vi "Ark Dino Leveler.vi"(8 "error in (no error)":errorcluster) -> (0 "error out":errorcluster)   [LabVIEW 2023]
uses:
  CTLs/Dump Stat.ctl
  <vilib>/Utility/config.llb/Config Data RefNum.ctl
  eb7943ba-f707-43d5-9dff-d1005f5da418.vi
  <vilib>/Utility/config.llb/Write Key (I32).vi
  <vilib>/Utility/inputDevices.llb/closeKeyboard.vi
  <vilib>/Utility/inputDevices.llb/closeMouse.vi
  <userlib>/_MGI/Application Control/MGI Gray if/MGI Gray if False.vi
  <vilib>/Utility/inputDevices.llb/keyboardAcquire.vi
  FaKI State Machine/FaKI State Machine.lvlib
  <vilib>/Utility/config.llb/NI_LVConfig.lvlib
panel:
  out "Application Hotkey":string
  in  "Delete Preset":bool
  in  "Select Monitor":i32=1 min=1 max=6
  in  "Start/Stop":bool
  in  "Dump Stat":T1
  out "Levels Remaining":i32
  in  "Levels Available":i32=85 min=0 max=1000
  in  "Save Preset":bool
  in  "Preset Name":string(combo)
  in  "No Oxy Stat?":bool
  in  "Levels":T2 {"HP" min=0 max=200; "Stamina" min=0 max=200; "Oxygen" min=0 max=200; "Food" min=0 max=200; "Weight" min=0 max=200; "Melee" min=0 max=200; "Speed" min=0 max=200}
  in  "Exit":bool
  # "(all remaining points go here)"
  # "(Golems, water tames, etc)"
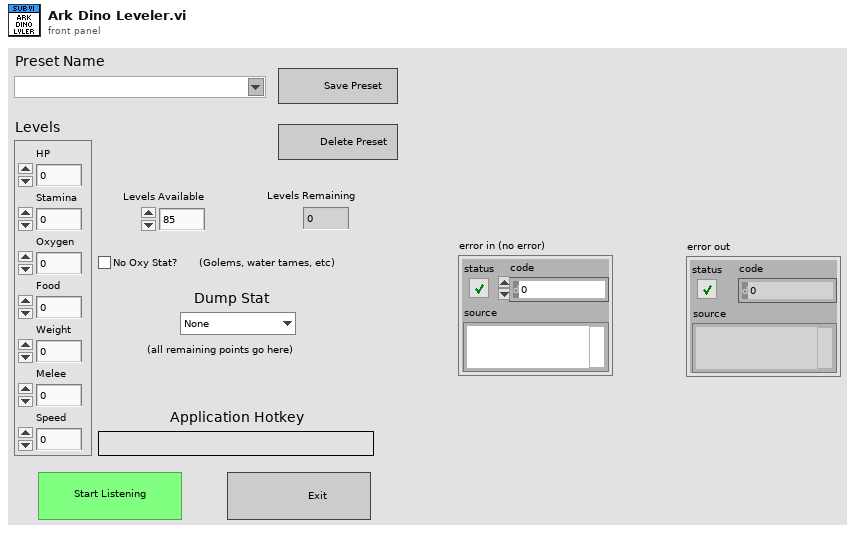
[diagram p1: front panel]
types:
  T1 = typedef "Dump Stat.ctl" = enum16{"None", "HP", "Stamina", "Oxygen", "Food", "Weight", "Melee", "Speed"}
  T2 = cluster{"HP":i32, "Stamina":i32, "Oxygen":i32, "Food":i32, "Weight":i32, "Melee":i32, "Speed":i32}
  T3 = enum8{"Enabled", "Disabled", "Disabled and Grayed Out"}
  T4 = enum32{"Invalid", "Standard", "Closed", "Hidden", "Minimized", "Maximized"}
  T5 = enum32{"invalid app kind", "Development System", "Run Time System", "Student Edition", "Embedded LabVIEW", "Evaluation", "Custom"}
  T6 = typedef "NI_LVConfig.lvlib/Config Data RefNum.ctl" = refnum<k1>
  T7 = cluster{"Core":cluster{"Current VI Reference":refnum<vi>, "Close Panel on Exit?":bool}, "Mouse":refnum<k1>, "Keyboard":refnum<k1>, "Config":T6, "Hotkey":enum16{"0", "1", "2", "3", "4", "5", "6", "7", "8", "9", "A", "B", "C", "D", "E", "F", "G", "H", "I", "J", "K", "L", "M", "N", "O", "P", "Q", "R", "S", "T", "U", "V", "W", "X", "Y", "Z", "F1", "F2", "F3", "F4", "F5", "F6", "F7", "F8", "F9", "F10", "F11", "F12", "F13", "F14", "F15", "ADD", "BACK", "BACKSLASH", "CAPITAL", "COMMA", "DECIMAL", "DELETE", "DIVIDE", "DOWN", "END", "EQUALS", "ESCAPE", "GRAVE (`)", "HOME", "INSERT", "LBRACKET", "LCONTROL", "LEFT", "L ALT", "LSHIFT", "LWIN", "MINUS", "MULTIPLY", "NEXT", "NUMLOCK", "NUMPAD_0", "NUMPAD_1", "NUMPAD_2", "NUMPAD_3", "NUMPAD_4", "NUMPAD_5", "NUMPAD_6", "NUMPAD_7", "NUMPAD_8", "NUMPAD_9", "PAUSE", "PERIOD", "PRIOR (PG UP)", "RBRACKET", "RCONTROL", "RETURN", "RIGHT", "R ALT", "RSHIFT", "RWIN", "SCROLL", "SEMICOLON", "SLASH", "SPACE", "SUBTRACT", "TAB", "UP", "ENTER (num pad)", "' (quote)"}[], "Res":cluster{"V":i16, "H":i16}[]}
  T8 = enum16{"0", "1", "2", "3", "4", "5", "6", "7", "8", "9", "A", "B", "C", "D", "E", "F", "G", "H", "I", "J", "K", "L", "M", "N", "O", "P", "Q", "R", "S", "T", "U", "V", "W", "X", "Y", "Z", "F1", "F2", "F3", "F4", "F5", "F6", "F7", "F8", "F9", "F10", "F11", "F12", "F13", "F14", "F15", "ADD", "BACK", "BACKSLASH", "CAPITAL", "COMMA", "DECIMAL", "DELETE", "DIVIDE", "DOWN", "END", "EQUALS", "ESCAPE", "GRAVE (`)", "HOME", "INSERT", "LBRACKET", "LCONTROL", "LEFT", "L ALT", "LSHIFT", "LWIN", "MINUS", "MULTIPLY", "NEXT", "NUMLOCK", "NUMPAD_0", "NUMPAD_1", "NUMPAD_2", "NUMPAD_3", "NUMPAD_4", "NUMPAD_5", "NUMPAD_6", "NUMPAD_7", "NUMPAD_8", "NUMPAD_9", "PAUSE", "PERIOD", "PRIOR (PG UP)", "RBRACKET", "RCONTROL", "RETURN", "RIGHT", "R ALT", "RSHIFT", "RWIN", "SCROLL", "SEMICOLON", "SLASH", "SPACE", "SUBTRACT", "TAB", "UP", "ENTER (num pad)", "' (quote)"}[]
  T9 = cluster{"Current VI Reference":refnum<vi>, "Close Panel on Exit?":bool}
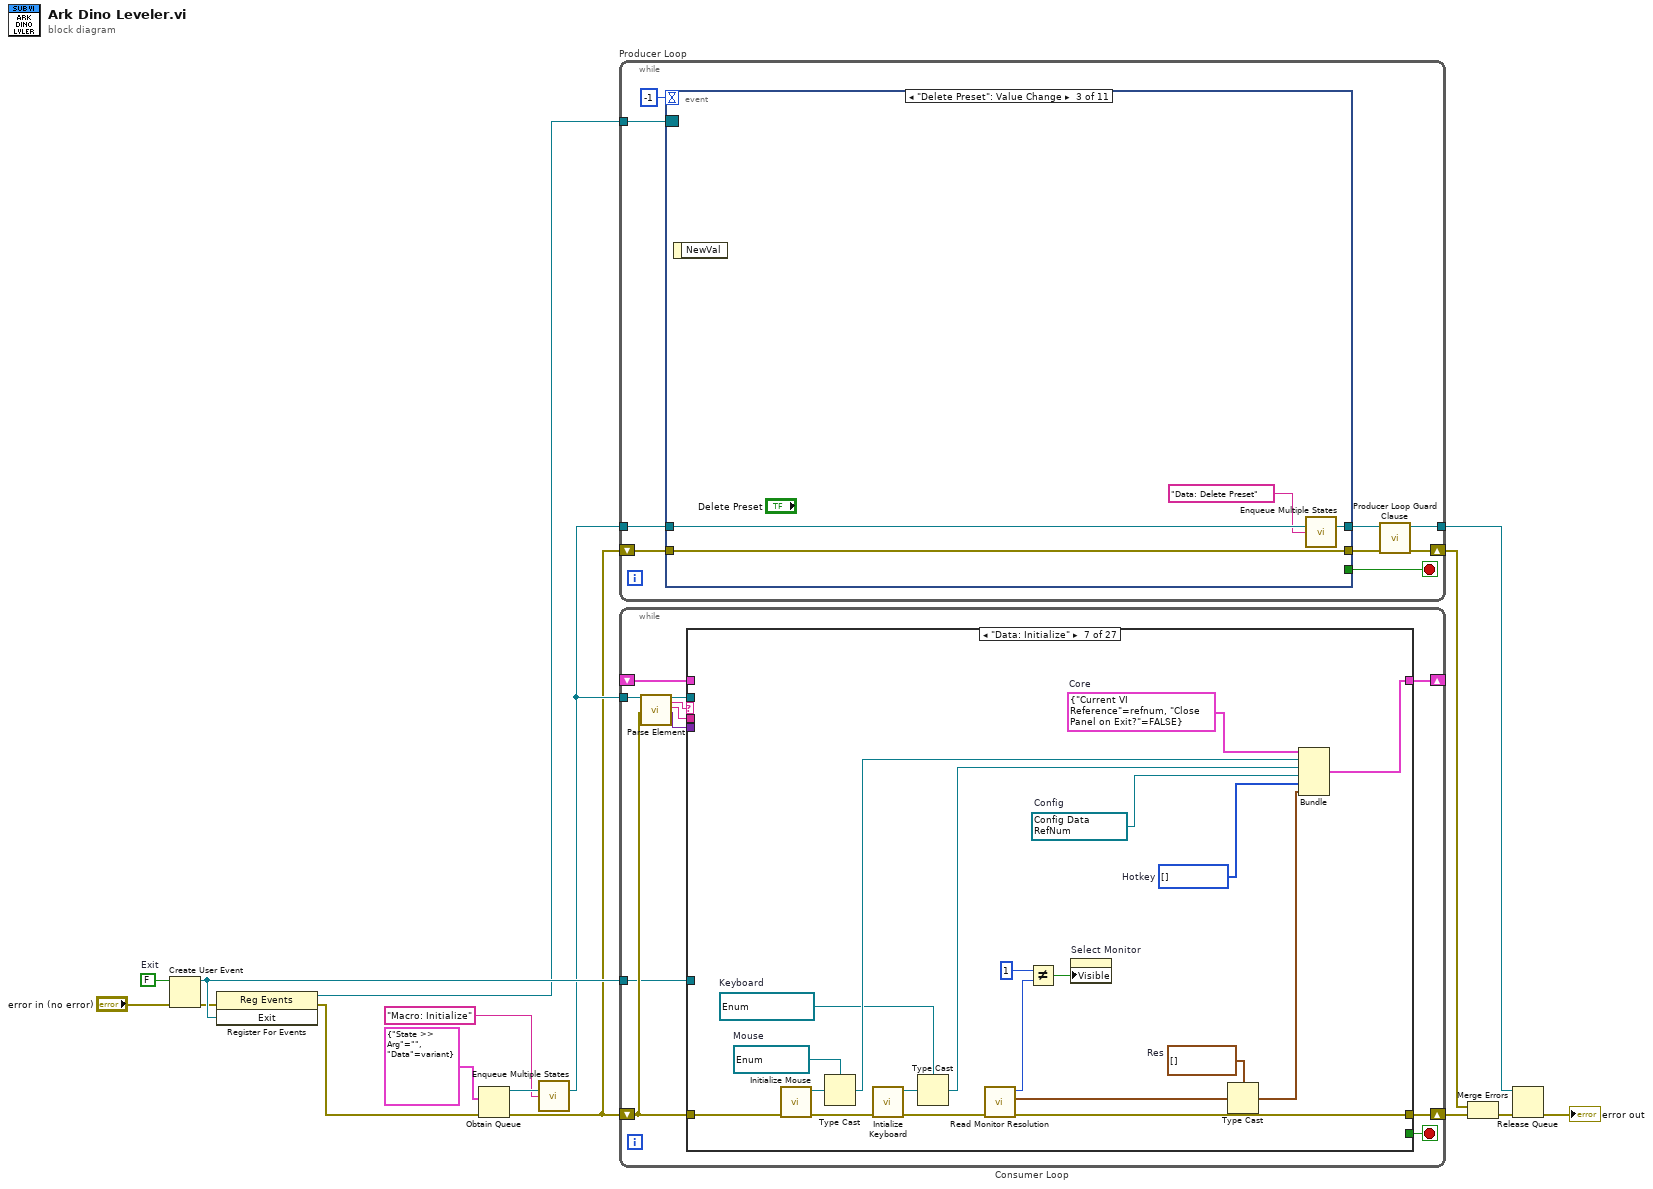
[diagram p0: block diagram]
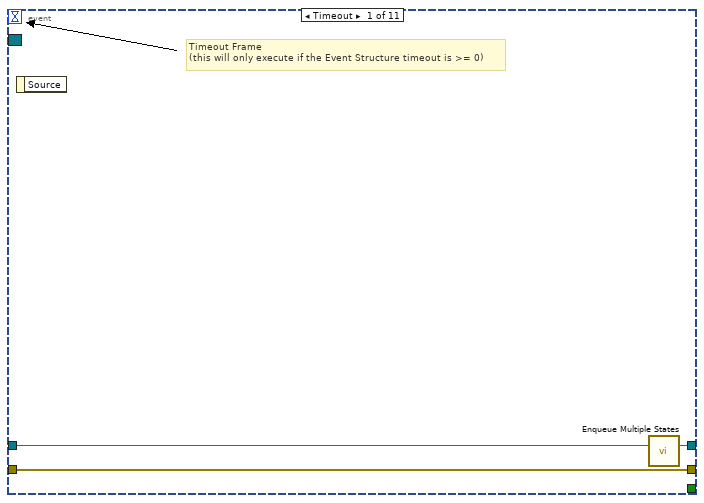
[diagram p2: hidden frame]
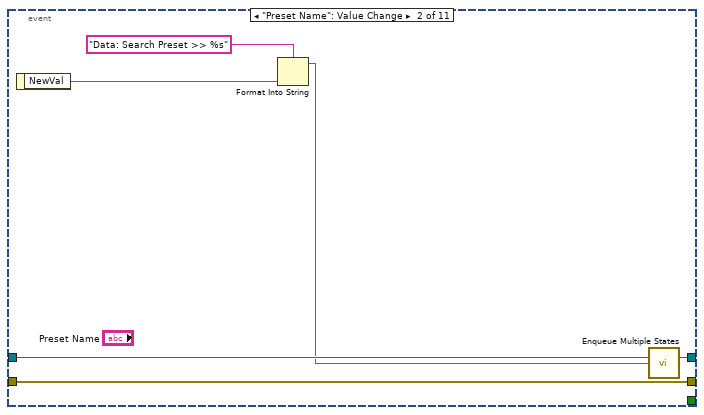
[diagram p3: hidden frame]
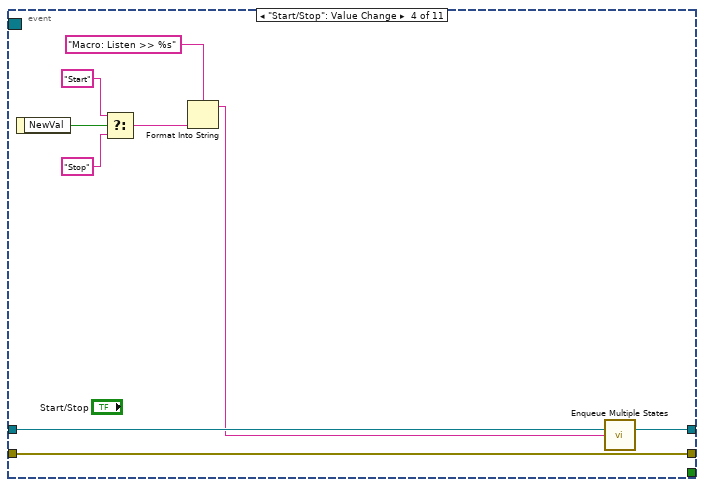
[diagram p4: hidden frame]
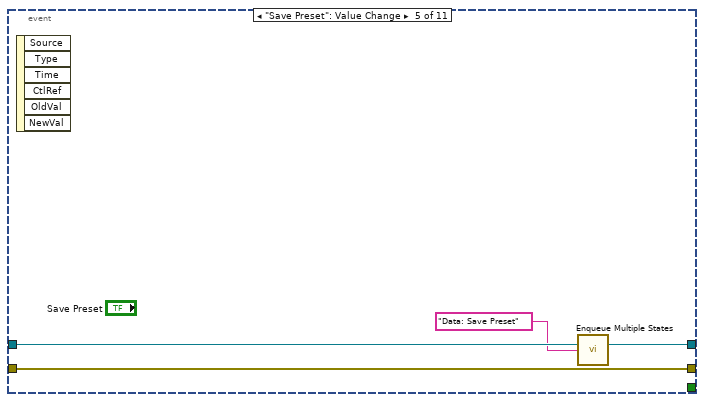
[diagram p5: hidden frame]
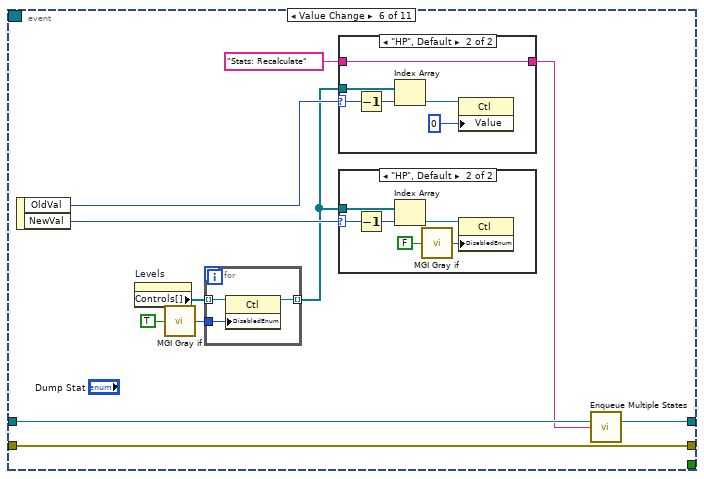
[diagram p6: hidden frame]
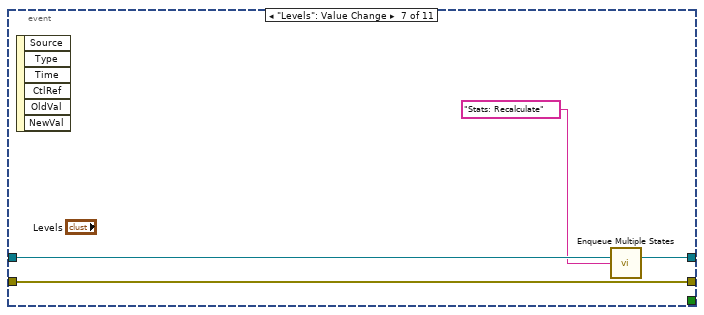
[diagram p9: hidden frame]
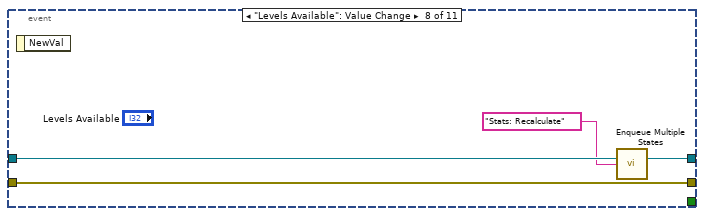
[diagram p10: hidden frame]
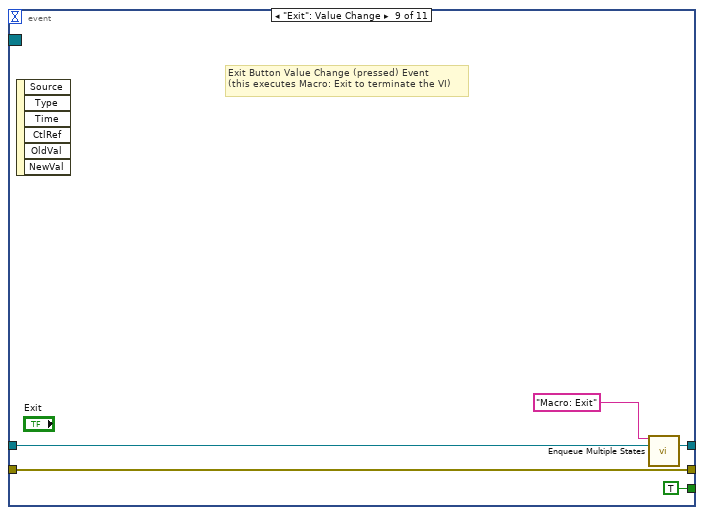
[diagram p11: hidden frame]
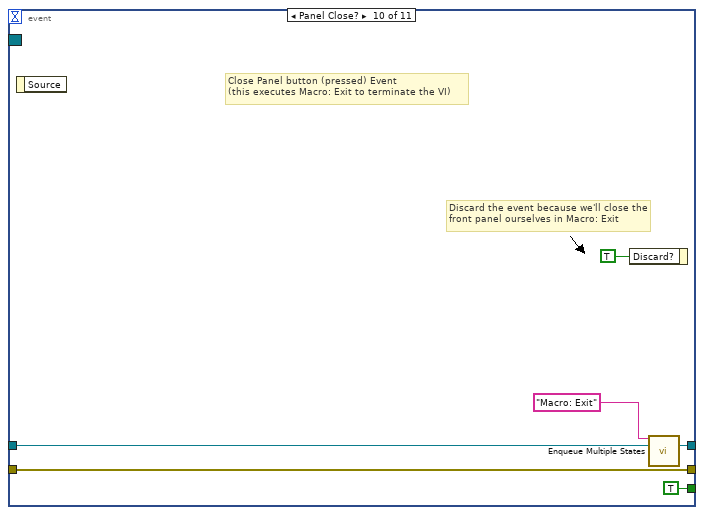
[diagram p12: hidden frame]
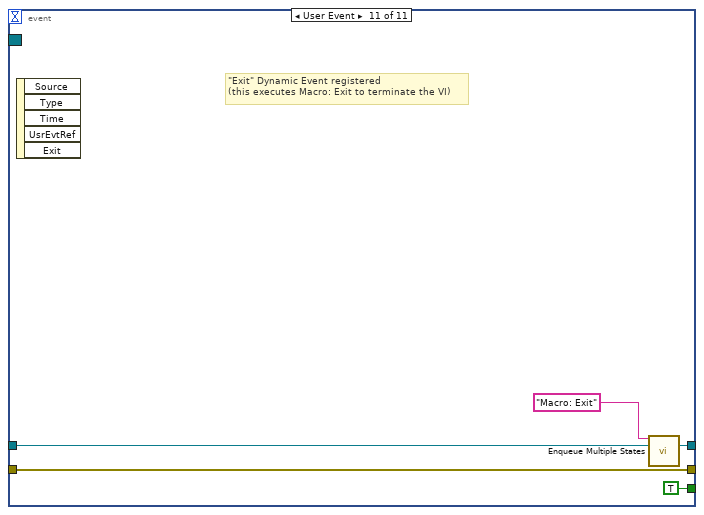
[diagram p13: hidden frame]
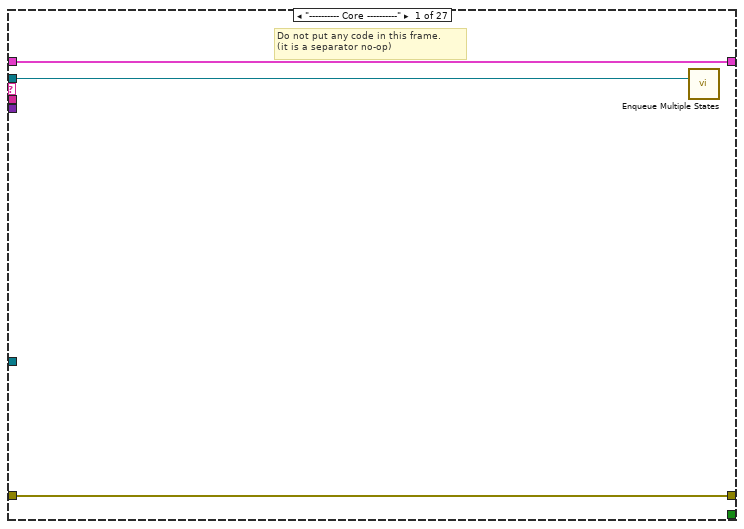
[diagram p14: hidden frame]
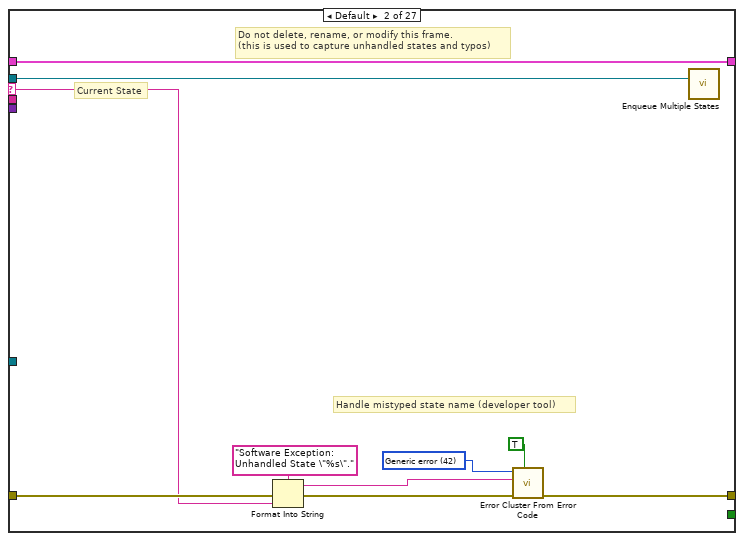
[diagram p15: hidden frame]
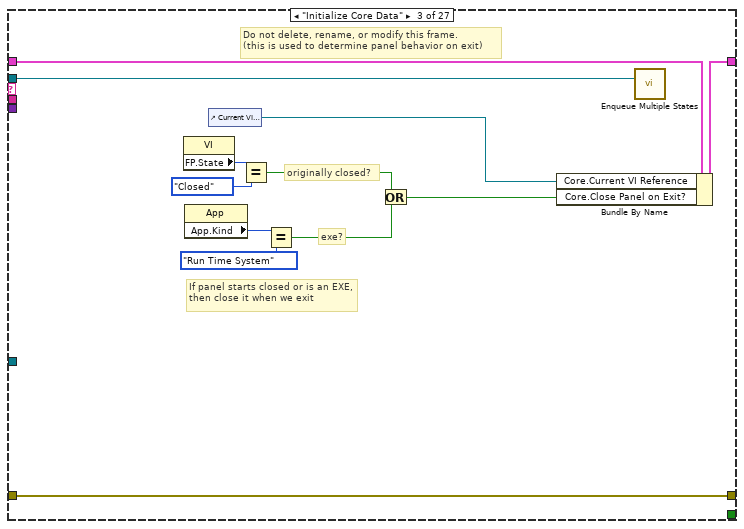
[diagram p16: hidden frame]
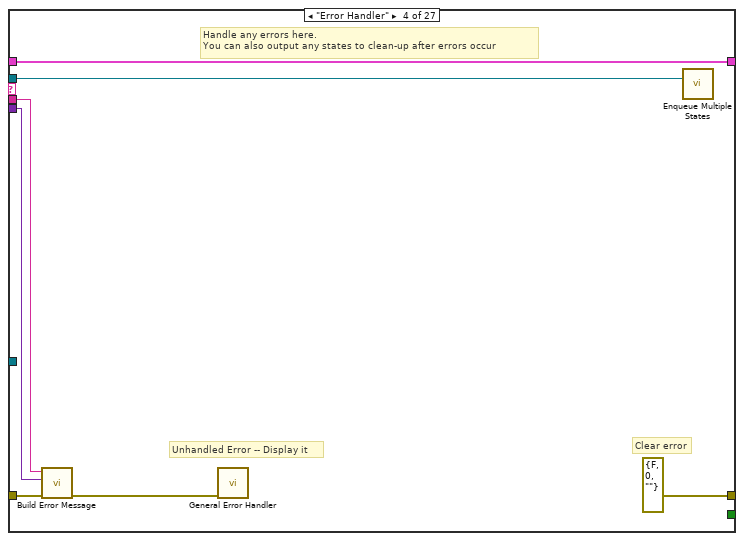
[diagram p17: hidden frame]
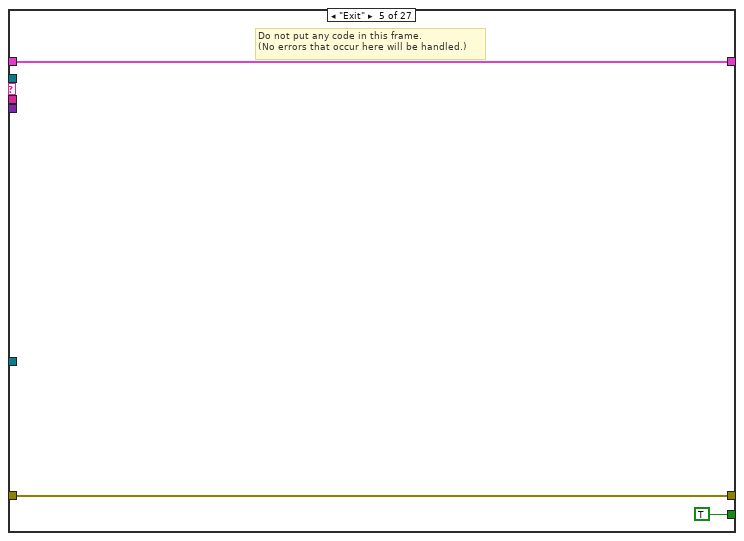
[diagram p18: hidden frame]
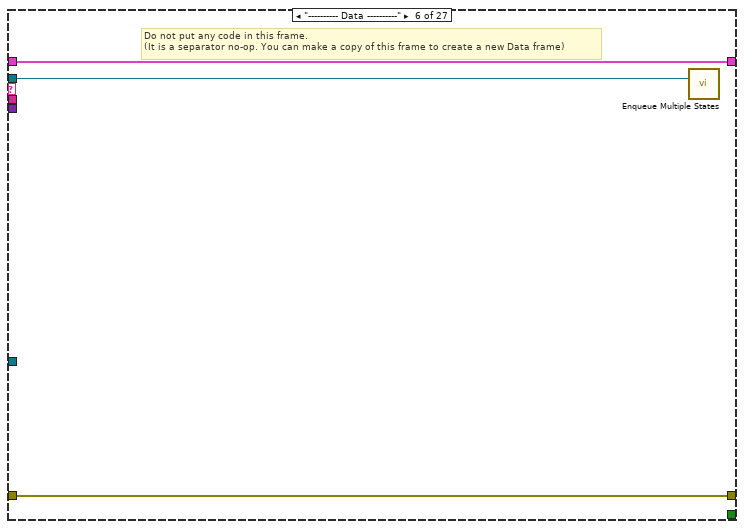
[diagram p19: hidden frame]
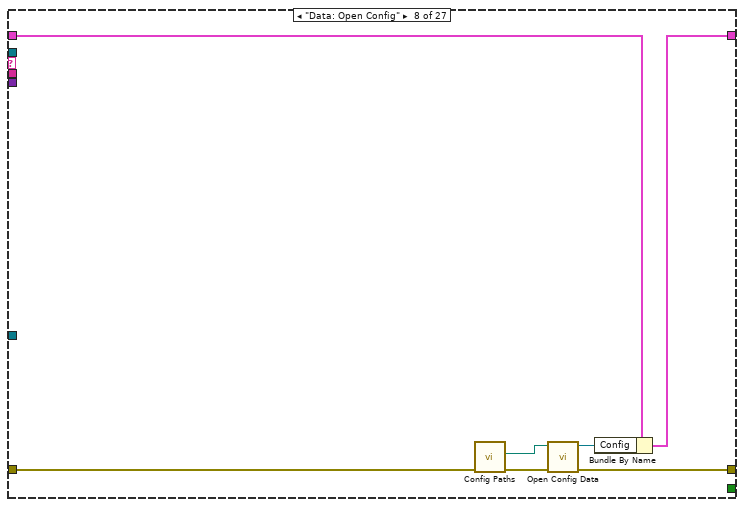
[diagram p20: hidden frame]
diagram:
  w13 = FALSE  # Exit
  n1 = Create User Event(user event datatype=w13, error in="error in (no error)") -> (user event=w16:refnum<user-event>, error out=w12:errorcluster)
  n2 = register-events(error in=w12, w16) -> (reference out=w15:refnum<event-registration>, error out=w14:errorcluster)  [unwired: 1 in]
  n3 = Obtain Queue(element data type=cluster{"State >> Arg":string, "Data":variant} {"State >> Arg"="", "Data"=variant}, error in (no error)=w14) -> (queue out=w6:refnum<queue>, error out=w3:errorcluster)  [unwired: 3 in, 1 out]
  n4 = call "Enqueue Multiple States.vi"("queue in"=w6, "State(s) at Back"="Macro: Initialize") -> ("queue out"=w7:refnum<queue>)  [unwired: 13 in]
  n5 = while "Producer Loop" {
    shift-right: [w20] -> w9
    shift-left: w3 -> [w25]
    tunnel: w15 -> [w17]
    tunnel: w7 -> [w23]
    tunnel: [w18] -> w11
    stop <- w22 stop-if-true
    n6 = event shown="[2] \"Delete Preset\": Value Change" {
      selector: w17 -> [_ _ _ _ _ _ _ _ _ _ _]
      dyn-events: _ -> [_ _ _ _ _ _ _ _ _ _ _]
      timeout: -1 ("Timeout") -> [_ _ _ _ _ _ _ _ _ _ _]
      tunnel: [w26 w32 w36 w47 w51 w62 w82 w86 w91 w97 w102] -> w21
      tunnel: w25 -> [w26 w32 w36 w47 w51 w62 w82 w86 w91 w97 w102]
      tunnel: w23 -> [w27 w33 w37 w43 w50 w53 w81 w85 w90 w94 w100]
      tunnel: [w28 w34 w38 w39 w49 w54 w80 w84 w88 w93 w99] -> w19
      tunnel: [_ _ _ _ _ _ _ _ TRUE TRUE TRUE] -> w22
      event Timeout {
        # "Timeout Frame\n(this will only execute if the Event Structure timeout is >= 0)"
        n7 = event-data() -> ()  [unwired: 1 in, 1 out]
        n8 = call "Enqueue Multiple States.vi"("queue in"=w27) -> ("queue out"=w28:refnum<queue>)  [unwired: 14 in]
      }
      event "Preset Name": Value Change {
        n9 = event-data() -> ("NewVal"=w30:string)  [unwired: 1 in]
        n10 = Format Into String(format string="Data: Search Preset >> %s" ("State(s) at Back"), w30) -> (resulting string=w29:string)  [unwired: 2 in, 1 out]
        n11 = call "Enqueue Multiple States.vi"("queue in"=w33, "State(s) at Back"=w29) -> ("queue out"=w34:refnum<queue>)  [unwired: 13 in]
      }
      event "Delete Preset": Value Change {
        n12 = event-data() -> ()  [unwired: 1 in, 1 out]
        n13 = call "Enqueue Multiple States.vi"("queue in"=w37, "State(s) at Back"="Data: Delete Preset") -> ("queue out"=w38:refnum<queue>)  [unwired: 13 in]
      }
      event "Start/Stop": Value Change {
        n14 = event-data() -> ("NewVal"=w44:bool)  [unwired: 1 in]
        n15 = Select(t="Start", s=w44, f="Stop") -> (s? t:f=w41:string)
        n16 = Format Into String(format string="Macro: Listen >> %s", w41) -> (resulting string=w40:string)  [unwired: 2 in, 1 out]
        n17 = call "Enqueue Multiple States.vi"("queue in"=w43, "State(s) at Back"=w40) -> ("queue out"=w39:refnum<queue>)  [unwired: 13 in]
      }
      event "Save Preset": Value Change {
        n18 = event-data() -> ()  [unwired: 1 in, 6 out]
        n19 = call "Enqueue Multiple States.vi"("queue in"=w50, "State(s) at Back"="Data: Save Preset") -> ("queue out"=w49:refnum<queue>)  [unwired: 13 in]
      }
      event Value Change {
        n20 = event-data() -> ("OldVal"=w57:T1, "NewVal"=w61:T1)  [unwired: 1 in]
        n21 = property on="Levels" class="Clust (strict)"() -> ("Controls[]"=w58:refnum<vi>[])  [unwired: 2 in, 2 out]
        n22 = call-poly <userlib>:"MGI Gray if.vi"("Boolean"=TRUE) -> ("Disabled"=w60:T3)
        n23 = for {
          tunnel: w58 -> [w72] mode=indexing
          tunnel: w60 -> [w71]
          tunnel: [w70] -> w56 mode=indexing
          n24 = property class="Ctl"(reference=w72, "DisabledEnum"=w71) -> (reference out=w70:refnum<vi>)  [unwired: 1 in, 1 out]
        }
        n25 = case shown="\"HP\", Default" w57 {
          selector: w57 -> [_ w69]
          tunnel: w56 -> [_ w68]
          tunnel: "Stats: Recalculate" -> [w63 w64]
          tunnel: [w63 w64] -> w52
          frame "None" {
          }
          frame "HP", Default {
            n26 = Decrement(x=w69) -> (x-1=w67:T1)
            n27 = Index Array(array=w68, index=w67) -> (element=w66:refnum<vi>)
            n28 = property class="Ctl"(reference=w66, "Value"=0 ("Select Monitor")) -> ()  [unwired: 1 in, 2 out]
          }
        }
        n29 = case shown="\"HP\", Default" w61 {
          selector: w61 -> [_ w78]
          tunnel: w56 -> [_ w75]
          frame "None" {
          }
          frame "HP", Default {
            n30 = Decrement(x=w78) -> (x-1=w74:T1)
            n31 = Index Array(array=w75, index=w74) -> (element=w73:refnum<vi>)
            n32 = call-poly <userlib>:"MGI Gray if.vi"("Boolean"=FALSE) -> ("Disabled"=w76:T3)
            n33 = property class="Ctl"(reference=w73, "DisabledEnum"=w76) -> ()  [unwired: 1 in, 2 out]
          }
        }
        n34 = call "Enqueue Multiple States.vi"("queue in"=w53, "State(s) at Back"=w52) -> ("queue out"=w54:refnum<queue>)  [unwired: 13 in]
      }
      event "Levels": Value Change {
        n35 = event-data() -> ()  [unwired: 1 in, 6 out]
        n36 = call "Enqueue Multiple States.vi"("queue in"=w81, "State(s) at Back"="Stats: Recalculate") -> ("queue out"=w80:refnum<queue>)  [unwired: 13 in]
      }
      event "Levels Available": Value Change {
        n37 = event-data() -> ()  [unwired: 1 in, 1 out]
        n38 = call "Enqueue Multiple States.vi"("queue in"=w85, "State(s) at Back"="Stats: Recalculate") -> ("queue out"=w84:refnum<queue>)  [unwired: 13 in]
      }
      event "Exit": Value Change {
        # "Exit Button Value Change (pressed) Event\n(this executes Macro: Exit to terminate the VI)"
        n39 = event-data() -> ()  [unwired: 1 in, 6 out]
        n40 = call "Enqueue Multiple States.vi"("State(s) at Front"="Macro: Exit", "queue in"=w90) -> ("queue out"=w88:refnum<queue>)  [unwired: 13 in]
      }
      event Panel Close? {
        # "Discard the event because we'll close the front panel ourselves in Macro: Exit"
        # "Close Panel button (pressed) Event\n(this executes Macro: Exit to terminate the VI)"
        n41 = event-data() -> ()  [unwired: 1 in, 1 out]
        n42 = event-data("Discard?"=TRUE) -> ()  [unwired: 1 in, 1 out]
        n43 = call "Enqueue Multiple States.vi"("State(s) at Front"="Macro: Exit", "queue in"=w94) -> ("queue out"=w93:refnum<queue>)  [unwired: 13 in]
      }
      event User Event {
        # "\"Exit\" Dynamic Event registered\n(this executes Macro: Exit to terminate the VI)"
        n44 = event-data() -> ()  [unwired: 1 in, 5 out]
        n45 = call "Enqueue Multiple States.vi"("State(s) at Front"="Macro: Exit", "queue in"=w100) -> ("queue out"=w99:refnum<queue>)  [unwired: 13 in]
      }
    }
    n46 = call "Producer Loop Guard Clause.vi"("error in (no error)"=w21, "queue in"=w19) -> ("error out"=w20:errorcluster, "queue out"=w18:refnum<queue>)  [unwired: 8 in]
  }
  n47 = while "Consumer Loop" {
    shift-right: [w110] -> _
    shift-left: _ -> [w109]
    shift-right: [w113] -> w8
    shift-left: w3 -> [w112]
    tunnel: w7 -> [w108]
    tunnel: w16 -> [w103]
    stop <- w111 stop-if-true
    n48 = call "Parse Element.vi"("queue in"=w108, "error in (no error)"=w112) -> ("queue out"=w107:refnum<queue>, "State"=w106:string, "Arg"=w105:string, "Data"=w104:variant)  [unwired: 14 in]
    n49 = case shown="\"Data: Initialize\"" w106 {
      selector: w106 -> [_ w118 _ _ _ _ _ _ _ _ _ _ _ _ _ _ _ _ _ _ _ _ _ _ _ _ _]
      tunnel: w107 -> [w114 w117 w127 w143 _ w149 _ _ w181 _ w202 _ _ w297 w300 w312 w316 w325 _ w407 w417 w420 w427 w434 w440 w450 _]
      tunnel: w105 -> [_ _ _ w139 _ _ _ _ _ w185 _ _ _ _ _ _ w317 w326 _ _ _ _ w426 _ _ _ _]
      tunnel: w109 -> [w115 w120 w133 w144 w147 w150 _ w178 w182 w190 w206 w256 w280 w294 w301 w304 w318 w328 w397 w416 w418 w422 w428 w438 w441 w451 w456]
      tunnel: [w116 w125 w138 errorcluster {"status"=FALSE, "code"=0, "source"=""} ("error out") w148 w151 w160 w175 w179 w183 w204 w253 w278 w295 w302 w310 w319 w329 w399 w413 w419 w423 w425 w439 w442 w452 w458] -> w113
      tunnel: w112 -> [w116 w124 w138 w142 w148 w151 w170 w174 w180 w191 w213 w263 w281 w299 w302 w311 w320 w330 w400 w414 w419 w423 w425 w439 w442 w452 w459]
      tunnel: [_ _ _ _ TRUE _ _ _ _ _ _ _ _ _ _ _ _ _ _ _ _ _ _ _ _ _ _] -> w111
      tunnel: [w115 w120 w137 w144 w147 w150 w166 w177 w182 w190 w203 w258 w280 w294 w301 w303 w318 w328 w397 w416 w418 w422 w428 w438 w441 w451 w456] -> w110
      tunnel: w104 -> [_ _ _ w140 _ _ _ _ _ _ _ _ _ _ _ _ _ _ _ _ _ _ _ _ _ _ _]
      tunnel: w103 -> [_ _ _ _ _ _ _ _ _ _ _ _ _ _ _ _ _ _ _ _ _ _ _ _ _ _ _]
      frame "---------- Core ----------" {
        # "Do not put any code in this frame.\n(it is a separator no-op)"
        n50 = call "Enqueue Multiple States.vi"("queue in"=w114) -> ()  [unwired: 14 in, 1 out]
      }
      frame Default {
        w122 = 42 items=["No error", "Argument error", "Memory is full", "Out of zone", "End of file", "File already open", "Generic file I/O error", "File not found", "File permission error", "Disk is full", "Duplicate path", "Too many files open", "System feature not enabled", "Resource file not found", "Cannot add resource", "Resource not found", "Image not found", "Image memory error", "Pen does not exist", "Config type invalid", "Config token not found", "Config parse error", "Config memory error", "Bad external code format", "Bad external code offset", "External code not present", "Null window", "Destroy window error", "Null menu", "Print aborted", "Bad print record", "Print driver error", "Windows error during printing", "Memory error during printing", "Print dialog error", "Generic print error", "Invalid device refnum", "Device not found", "Device parameter error", "Device unit error", "Cannot open device", "Device call aborted", "Generic error", "Cancelled by user", "Object ID too low", "Object ID too high", "Object not in heap", "Unknown heap", "Unknown object (invalid DefProc)", "Unknown object (DefProc not in table)", "Message out of range", "Invalid (null) method", "Unknown message", "Manager call not supported", "Bad address", "Network operation in progress", "Network operation timed out", "Connection is busy", "Network attribute not supported", "Network error", "Address in use", "System out of memory", "Connection aborted", "Connection refused", "Not connected", "Already connected", "Connection closed", "Initialization error (interapplication manager)", "Bad occurrence", "Wait on unbound occurrence handler", "Occurrence queue overflow", "Datalog type conflict", "Unused", "Unrecognized type (interapplication manager)", "Memory corrupt", "Failed to make temporary DLL", "Old CIN version", "Drag socket not found", "Failed to load drop-object", "Failed to register OLE object", "Failed to release OLE object", "Format specifier type mismatch", "Unknown format specifier", "Too few format specifiers", "Too many format specifiers", "Scan failed", "Newer CIN version", "Error converting to variant", "Runtime menu error", "Password tampered", "Variant attribute not found", "Incompatible variant data type", "Event data is not available", "Event Store is not present", "Occurrence is not found", "Event Queue is not created", "Event info is not available", "Refnum passed is NULL", "Error retrieving Class GUID", "Error retrieving CoClass GUID", "Error retrieving TypeLib GUID.", "Bad built application magic bytes.", "Specific driver is different from the specific driver associated with the Logical Name.", "There is no session opened to the class driver.", "Max Error", "MAX - Error with config objects", "MAX - Error loading configuration", "MAX - Group not supported"]
        # "Current State"
        # "Do not delete, rename, or modify this frame.\n(this is used to capture unhandled states and typos)"
        # "Handle mistyped state name (developer tool)"
        n51 = Format Into String(format string="Software Exception: Unhandled State \"%s\"." ("message"), error in=w124, w118) -> (resulting string=w121:string, error out=w126:errorcluster)  [unwired: 1 in]
        n52 = call <vilib>:"Error Cluster From Error Code.vi"("show call chain? (False)"=TRUE, "error in (no error)"=w126, "error message (\"\")"=w121, "error code (0)"=w122) -> ("error out"=w125:errorcluster)  [unwired: 5 in]
        n53 = call "Enqueue Multiple States.vi"("queue in"=w117) -> ()  [unwired: 14 in, 1 out]
      }
      frame "Initialize Core Data" {
        # "Do not delete, rename, or modify this frame.\n(this is used to determine panel behavior on exit)"
        # "originally closed?"
        # "exe?"
        # "If panel starts closed or is an EXE, then close it when we exit"
        n54 = property class="VI"() -> ("FP.State"=w130:T4)  [unwired: 2 in, 2 out]
        n55 = property class="App"() -> ("App.Kind"=w136:T5)  [unwired: 2 in, 2 out]
        n56 = control-ref of="Current VI Reference"() -> (w131:refnum<vi>)
        n57 = Equal?(x=w130, y=T4."Closed" ("Front Panel Window:State")) -> (x = y?=w128:bool)
        n58 = Equal?(x=w136, y=T5."Run Time System" ("Application:Kind")) -> (x = y?=w134:bool)
        n59 = Or(x=w128, y=w134) -> (x .or. y?=w132:bool)
        n60 = Bundle By Name(cluster=w133, "Core.Current VI Reference"=w131, "Core.Close Panel on Exit?"=w132) -> (w137:T7)
        n61 = call "Enqueue Multiple States.vi"("queue in"=w127) -> ()  [unwired: 14 in, 1 out]
      }
      frame "Error Handler" {
        # "Unhandled Error -- Display it"
        # "Handle any errors here.\nYou can also output any states to clean-up after errors occur"
        # "Clear error"
        n62 = call "Build Error Message.vi"("error in (no error)"=w142, "Data"=w140, "Arg"=w139) -> ("error out"=w141:errorcluster)  [unwired: 8 in]
        n63 = call <vilib>:"General Error Handler.vi"("error in (no error)"=w141) -> ()  [unwired: 10 in, 5 out]
        n64 = call "Enqueue Multiple States.vi"("queue in"=w143) -> ()  [unwired: 14 in, 1 out]
      }
      frame "Exit" {
        # "Do not put any code in this frame.\n(No errors that occur here will be handled.)"
      }
      frame "---------- Data ----------" {
        # "Do not put any code in this frame.\n(It is a separator no-op. You can make a copy of this frame to create a new Data frame)"
        n65 = call "Enqueue Multiple States.vi"("queue in"=w149) -> ()  [unwired: 14 in, 1 out]
      }
      frame "Data: Initialize" {
        w152 = T8 [] items=["0", "1", "2", "3", "4", "5", "6", "7", "8", "9", "A", "B", "C", "D", "E", "F", "G", "H", "I", "J", "K", "L", "M", "N", "O", "P", "Q", "R", "S", "T", "U", "V", "W", "X", "Y", "Z", "F1", "F2", "F3", "F4", "F5", "F6", "F7", "F8", "F9", "F10", "F11", "F12", "F13", "F14", "F15", "ADD", "BACK", "BACKSLASH", "CAPITAL", "COMMA", "DECIMAL", "DELETE", "DIVIDE", "DOWN", "END", "EQUALS", "ESCAPE", "GRAVE (`)", "HOME", "INSERT", "LBRACKET", "LCONTROL", "LEFT", "L ALT", "LSHIFT", "LWIN", "MINUS", "MULTIPLY", "NEXT", "NUMLOCK", "NUMPAD_0", "NUMPAD_1", "NUMPAD_2", "NUMPAD_3", "NUMPAD_4", "NUMPAD_5", "NUMPAD_6", "NUMPAD_7", "NUMPAD_8", "NUMPAD_9", "PAUSE", "PERIOD", "PRIOR (PG UP)", "RBRACKET", "RCONTROL", "RETURN", "RIGHT", "R ALT", "RSHIFT", "RWIN", "SCROLL", "SEMICOLON", "SLASH", "SPACE", "SUBTRACT", "TAB", "UP", "ENTER (num pad)", "' (quote)"]  # Hotkey
        w153 = T6 refnum items=["config data"]  # Config
        w158 = cluster{"V":i16, "H":i16}[] []  # Res
        w163 = refnum<k1> refnum items=["KEYBOARD"]  # Keyboard
        w167 = refnum<k1> refnum items=["MOUSE"]  # Mouse
        w171 = T9 {"Current VI Reference"=refnum, "Close Panel on Exit?"=FALSE}  # Core
        n66 = call <vilib>:"Initialize Mouse.vi"("error in (no error)"=w170) -> ("error out"=w169:errorcluster, "device ID"=w168:refnum<k1>)  [unwired: 9 in]
        n67 = Type Cast(type=w167, x=w168) -> (*(type *) &x=w164:refnum<k1>)
        n68 = call <vilib>:"Intialize Keyboard.vi"("error in (no error)"=w169) -> ("error out"=w161:errorcluster, "device ID"=w165:refnum<k1>)  [unwired: 9 in]
        n69 = Type Cast(type=w163, x=w165) -> (*(type *) &x=w162:refnum<k1>)
        n70 = call "Read Monitor Resolution.vi"("error in (no error)"=w161) -> ("error out"=w160:errorcluster, "Monitor Resolution"=w159:cluster{"H":i16, "V":i16}[], "Number of Displays"=w157:i32)  [unwired: 8 in]
        n71 = Not Equal?(x=1, y=w157) -> (x != y?=w155:bool)
        n72 = property on="Select Monitor" class="DigNum (strict)"("Visible"=w155) -> ()  [unwired: 2 in, 2 out]
        n73 = Type Cast(type=w158, x=w159) -> (*(type *) &x=w154:cluster{"V":i16, "H":i16}[])
        n74 = Bundle("Core"=w171, "Mouse"=w164, "Keyboard"=w162, "Config"=w153, "Hotkey"=w152, "Res"=w154) -> (w166:T7)  [unwired: 1 in]
      }
      frame "Data: Open Config" {
        n75 = call "Config Paths.vi"("error in (no error)"=w174) -> ("error out"=w173:errorcluster, "Preset Config"=w172:path)  [unwired: 7 in, 2 out]
        n76 = call <vilib>:"Open Config Data.vi"("error in (no error)"=w173, "configuration file path"=w172) -> ("error out"=w175:errorcluster, "refnum"=w176:T6)  [unwired: 7 in, 1 out]
        n77 = Bundle By Name(cluster=w178, "Config"=w176) -> (w177:T7)
      }
      frame "Data: Flush Queue" {
        n78 = Flush Queue(queue=w181, error in (no error)=w180) -> (error out=w179:errorcluster)  [unwired: 2 out]
      }
      frame "Data: Search Preset" {
        n79 = Unbundle By Name(w190) -> ("Config"=w189:T6)
        n80 = call <vilib>:"Get Section Names.vi"("error in (no error)"=w191, "refnum"=w189) -> ("error out"=w186:errorcluster, "section names"=w188:string[], "refnum out"=w184:T6)  [unwired: 7 in]
        n81 = Search 1D Array(1D array=w188, element=w185) -> (index of element=w187:i32)  [unwired: 1 in]
        n82 = case shown="0, Default" w187 {
          tunnel: w186 -> [w199 w200]
          tunnel: w185 -> [w198 _]
          tunnel: w184 -> [w197 _]
          tunnel: [w196 w200] -> w183
          frame 0, Default {
            n83 = call "Load Preset.vi"("error in (no error)"=w199, "Preset Name"=w198, "Config"=w197) -> ("error out"=w196:errorcluster, "Dump Stat"=w192:T1, "Levels Available"=w193:i32, "Levels"=w194:T2, "No Oxy?"=w195:bool)  [unwired: 4 in]
            n84 = property on="No Oxy Stat?" class="Bool (strict)"("Val(Sgnl)"=w195) -> ()  [unwired: 2 in, 2 out]
            n85 = property on="Levels" class="Clust (strict)"("Val(Sgnl)"=w194) -> ()  [unwired: 2 in, 2 out]
            n86 = property on="Levels Available" class="DigNum (strict)"("Val(Sgnl)"=w193) -> ()  [unwired: 2 in, 2 out]
            n87 = property on="Dump Stat" class="Enum (strict)"("Val(Sgnl)"=w192) -> ()  [unwired: 2 in, 2 out]
          }
          frame -1 {
          }
        }
      }
      frame "Data: Save Preset" {
        # "in case a new preset was saved,\nneed to add that to list of names"
        n88 = local read "Preset Name"() -> (w208:string)
        n89 = Unbundle By Name(w206) -> ("Config"=w212:T6)
        n90 = call <vilib>:"Get Section Names.vi"("error in (no error)"=w213, "refnum"=w212) -> ("error out"=w209:errorcluster, "section names"=w211:string[])  [unwired: 7 in, 1 out]
        n91 = Search 1D Array(1D array=w211, element=w208) -> (index of element=w210:i32)  [unwired: 1 in]
        n92 = case shown="0, Default" w210 {
          tunnel: w209 -> [w231 w232]
          tunnel: [w230 w232] -> w205
          tunnel: [w229 TRUE ("Overwrite")] -> w207
          frame 0, Default {
            n93 = call "Overwrite?"("error in (no error)"=w231) -> ("error out"=w230:errorcluster, "Overwrite"=w229:bool)  [unwired: 9 in]
          }
          frame -1 {
          }
        }
        n94 = case shown="True" w207 {
          tunnel: w206 -> [w214 w219]
          tunnel: w205 -> [w215 w218]
          tunnel: [w215 w217] -> w204
          tunnel: [w214 w216] -> w203
          frame False {
          }
          frame True {
            n95 = in-place {
              in-place-border: w218 -> [w226]
              in-place-border: [w225] -> w217
              n96 = in-place-cluster #1(w219) -> ("Config"=w228:T6)
              n97 = local read "Levels Available"() -> (w221:i32)
              n98 = local read "No Oxy Stat?"() -> (w223:bool)
              n99 = local read "Preset Name"() -> (w224:string)
              n100 = local read "Dump Stat"() -> (w220:T1)
              n101 = local read "Levels"() -> (w222:T2)
              n102 = call "Save Preset.vi"("No Oxy?"=w223, "Dump Stat"=w220, "Preset Name"=w224, "error in (no error)"=w226, "Levels Available"=w221, "Levels"=w222, "Config"=w228) -> ("error out"=w225:errorcluster, "Config out"=w227:T6)  [unwired: 3 in]
              n103 = in-place-cluster #1("Config"=w227) -> (w216:T7)
            }
          }
        }
        n104 = call "Enqueue Multiple States.vi"("queue in"=w202, "State(s) at Back"="UI: Get Preset Names") -> ()  [unwired: 13 in, 1 out]
      }
      frame "Data: Save Preset old" {
        w251 = refnum<vi> refnum  # Numeric
        n105 = local read "Levels Available"() -> (w244:i32)
        n106 = local read "No Oxy Stat?"() -> (w246:bool)
        n107 = property on="Levels" class="Clust (strict)"() -> ("Controls[]"=w252:refnum<vi>[])  [unwired: 2 in, 2 out]
        n108 = Unbundle By Name(w256) -> ("Config"=w255:T6)
        n109 = local read "Dump Stat"() -> (w242:T1)
        n110 = local read "Preset Name"() -> (w254:string)
        n111 = for {
          tunnel: w252 -> [w276] mode=indexing
          tunnel: w251 -> [w275]
          tunnel: [w273] -> w250 mode=indexing
          tunnel: [w272] -> w247 mode=indexing
          n112 = To More Specific Class(target class=w275, reference=w276) -> (specific class reference=w274:refnum<vi>)  [unwired: 1 in, 1 out]
          n113 = property class="Num"(reference=w274) -> ("Label.Text"=w272:string, "Value"=w273:variant)  [unwired: 1 in, 2 out]
        }
        n114 = Boolean To (0,1)(Boolean=w246) -> (0, 1=w240:i16)
        n115 = Bundle By Name(cluster=cluster{"Label.Text":string, "Numeric":i32} {"Label.Text"="DumpStat", "Numeric"=0}, "Numeric"=w242) -> (w238:cluster{"Label.Text":string, "Numeric":i32})
        n116 = Bundle By Name(cluster=cluster{"Label.Text":string, "Numeric":i32} {"Label.Text"="LevelsAvailable", "Numeric"=0}, "Numeric"=w244) -> (w237:cluster{"Label.Text":string, "Numeric":i32})
        n117 = Bundle By Name(cluster=cluster{"Label.Text":string, "Numeric":i32} {"Label.Text"="NoOxy?", "Numeric"=0}, "Numeric"=w240) -> (w239:cluster{"Label.Text":string, "Numeric":i32})
        n118 = Build Array(w237, w238, w239) -> (w235:cluster{"Label.Text":string, "Numeric":i32}[])
        n119 = Variant To Data(type=i32[] [], Variant=w250) -> (data=w248:i32[])  [unwired: 1 in, 1 out]
        n120 = Build Cluster Array(w247, w248) -> (w236:cluster{"Label.Text":string, "Numeric":i32}[])
        n121 = Insert Into Array(array=w236, new element=w235) -> (w234:cluster{"Label.Text":string, "Numeric":i32}[])  [unwired: 1 in]
        n122 = for {
          tunnel: w254 -> [w267]
          shift-right: [w269] -> w261
          shift-left: w263 -> [w271]
          tunnel: w234 -> [w266] mode=indexing
          shift-right: [w270] -> w262
          shift-left: w255 -> [w268]
          n123 = Unbundle(w266) -> ("Label.Text"=w264:string, "Numeric"=w265:i32)
          n124 = call-poly <vilib>:"Write Key.vi"("section"=w267, "error in (no error)"=w271, "value"=w265, "key"=w264, "refnum"=w268) -> ("error out"=w269:errorcluster, "refnum out"=w270:T6)  [unwired: 4 in, 1 out]
        }
        n125 = call <vilib>:"Close Config Data.vi"("error in (no error)"=w261, "refnum"=w262) -> ("error out"=w259:errorcluster, "file path"=w260:path)  [unwired: 8 in]
        n126 = call <vilib>:"Open Config Data.vi"("error in (no error)"=w259, "configuration file path"=w260) -> ("error out"=w253:errorcluster, "refnum"=w257:T6)  [unwired: 7 in, 1 out]
        n127 = Bundle By Name(cluster=w256, "Config"=w257) -> (w258:T7)
      }
      frame "Data: Delete Preset" {
        n128 = call "Perm Delete?"("error in (no error)"=w281) -> ("error out"=w279:errorcluster, "Delete"=w277:bool)  [unwired: 9 in]
        n129 = case shown="True" w277 {
          tunnel: w280 -> [_ w289]
          tunnel: w279 -> [w282 w288]
          tunnel: [w282 w283] -> w278
          frame False {
          }
          frame True {
            n130 = Unbundle By Name(w289) -> ("Config"=w287:T6)
            n131 = local read "Preset Name"() -> (w286:string)
            n132 = call <vilib>:"Remove Section.vi"("section"=w286, "error in (no error)"=w288, "refnum"=w287) -> ("error out"=w284:errorcluster)  [unwired: 6 in, 2 out]
            n133 = property on="Preset Name" class="CmbBox"(error in=w284, "Val(Sgnl)"="") -> (error out=w283:errorcluster)  [unwired: 1 in, 1 out]
          }
        }
      }
      frame "Data: Cleanup" {
        # "Cleanup any data and references, here.\n(this is called automatically, by the Macro: Exit)"
        n134 = Unbundle By Name(w294) -> ("Core.Current VI Reference"=w298:refnum<vi>)
        n135 = Unbundle By Name(w294) -> ("Mouse"=w292:refnum<k1>, "Keyboard"=w293:refnum<k1>)
        n136 = Close Reference(reference=w298, error in (no error)=w299) -> (error out=w291:errorcluster)
        n137 = invoke class="VI" method="Default Vals.Reinit All"(error in=w291) -> (error out=w290:errorcluster)  [unwired: 2 in, 2 out]
        n138 = call-poly <vilib>:"Close Input Device.vi"("error in (no error)"=w290, "device ID"=w293) -> ("error out"=w296:errorcluster)  [unwired: 8 in]
        n139 = call-poly <vilib>:"Close Input Device.vi"("error in (no error)"=w296, "device ID"=w292) -> ("error out"=w295:errorcluster)  [unwired: 8 in]
        n140 = call "Enqueue Multiple States.vi"("queue in"=w297) -> ()  [unwired: 14 in, 1 out]
      }
      frame "---------- UI ----------" {
        # "Do not put any code in this frame.\n(It is a separator no-op. You can make a copy of this frame to create a new UI frame)"
        n141 = call "Enqueue Multiple States.vi"("queue in"=w300) -> ()  [unwired: 14 in, 1 out]
      }
      frame "UI: Initialize" {
        # "Initialize the User Interface, here.\n(this is called automatically, by the Macro: Init)"
        n142 = call "Hotkey FGV.vi"("error in (no error)"=w311) -> ("error out"=w310:errorcluster, "Hotkey String out"=→"Application Hotkey":string, "Hotkey out"=w305:T8)  [unwired: 8 in]
        n143 = property on="Levels" class="Clust (strict)"() -> ("Controls[]"=w307:refnum<vi>[])  [unwired: 2 in, 2 out]
        n144 = call-poly <userlib>:"MGI Gray if.vi"("Boolean"=TRUE) -> ("Disabled"=w308:T3)
        n145 = for {
          tunnel: w307 -> [w315] mode=indexing
          tunnel: w308 -> [w314]
          tunnel: [w313] -> _ mode=indexing
          n146 = property class="Ctl"(reference=w315, "DisabledEnum"=w314) -> (reference out=w313:refnum<vi>)  [unwired: 1 in, 1 out]
        }
        n147 = Bundle By Name(cluster=w304, "Hotkey"=w305) -> (w303:T7)
        n148 = call "Enqueue Multiple States.vi"("queue in"=w312) -> ()  [unwired: 14 in, 1 out]
      }
      frame "UI: Cursor Set" {
        # "Argument"
        # "Set and Unset Cursor Busy.\n(Usage: \"UI: Cursor Set >> Busy|Idle\")"
        n149 = case shown="\"Idle\", Default" w317 {
          tunnel: w320 -> [w322 w324]
          tunnel: [w321 w323] -> w319
          frame "Idle", Default {
            n150 = call <vilib>:"Unset Busy.vi"("error in (no error)"=w322) -> ("error out"=w321:errorcluster)  [unwired: 10 in]
          }
          frame "Busy" {
            n151 = call <vilib>:"Set Busy.vi"("error in (no error)"=w324) -> ("error out"=w323:errorcluster)  [unwired: 9 in, 1 out]
          }
        }
        n152 = call "Enqueue Multiple States.vi"("queue in"=w316) -> ()  [unwired: 14 in, 1 out]
      }
      frame "UI: Front Panel State" {
        # "Argument"
        # "Set Front Panel Open or Closed\n(Usage: \"UI: Front Panel State >> Open|Close\")"
        n153 = Unbundle By Name(w328) -> ("Core.Current VI Reference"=w327:refnum<vi>)
        n154 = case shown="\"Open\", \"Standard\", Default" w326 {
          tunnel: w330 -> [w337 w351 w363 w376 w389]
          tunnel: [w338 w352 w364 w377 w390] -> w329
          tunnel: w327 -> [w335 w349 w361 w374 w387]
          frame "Open", "Standard", Default {
            w331 = T4."Standard" ("State")
            n155 = property class="VI"(reference=w335, error in=w337) -> (reference out=w334:refnum<vi>, error out=w336:errorcluster, "FP.State"=w333:T4)
            n156 = Not Equal?(x=w333, y=w331) -> (x != y?=w332:bool)
            n157 = case shown="True" w332 {
              tunnel: [w343 w344] -> w338
              tunnel: w336 -> [w342 w344]
              tunnel: w334 -> [w340 _]
              tunnel: w331 -> [w339 _]
              frame True {
                n158 = invoke class="VI" method="FP.Open"(reference=w340, error in=w342, "Activate"=TRUE, "State"=w339) -> (error out=w343:errorcluster)  [unwired: 1 in, 4 out]
              }
              frame False {
              }
            }
          }
          frame "Close", "Closed" {
            n159 = property class="VI"(reference=w349, error in=w351) -> (reference out=w348:refnum<vi>, error out=w350:errorcluster, "FP.State"=w346:T4)
            n160 = Not Equal?(x=w346, y=T4."Closed" ("Front Panel Window:State")) -> (x != y?=w345:bool)
            n161 = case shown="True" w345 {
              tunnel: [w353 w356] -> w352
              tunnel: w350 -> [w353 w355]
              tunnel: w348 -> [_ w354]
              frame False {
              }
              frame True {
                n162 = invoke class="VI" method="FP.Close"(reference=w354, error in=w355) -> (error out=w356:errorcluster)  [unwired: 1 in, 2 out]
              }
            }
          }
          frame "Hidden", "Hide" {
            w357 = T4."Hidden" ("State")
            n163 = property class="VI"(reference=w361, error in=w363) -> (reference out=w360:refnum<vi>, error out=w362:errorcluster, "FP.State"=w359:T4)
            n164 = Not Equal?(x=w359, y=w357) -> (x != y?=w358:bool)
            n165 = case shown="True" w358 {
              tunnel: [w368 w369] -> w364
              tunnel: w362 -> [w367 w369]
              tunnel: w360 -> [w366 _]
              tunnel: w357 -> [w365 _]
              frame True {
                n166 = invoke class="VI" method="FP.Open"(reference=w366, error in=w367, "State"=w365) -> (error out=w368:errorcluster)  [unwired: 2 in, 4 out]
              }
              frame False {
              }
            }
          }
          frame "Minimize", "Minimized" {
            w370 = T4."Minimized" ("State")
            n167 = property class="VI"(reference=w374, error in=w376) -> (reference out=w373:refnum<vi>, error out=w375:errorcluster, "FP.State"=w372:T4)
            n168 = Not Equal?(x=w372, y=w370) -> (x != y?=w371:bool)
            n169 = case shown="True" w371 {
              tunnel: [w381 w382] -> w377
              tunnel: w375 -> [w380 w382]
              tunnel: w373 -> [w379 _]
              tunnel: w370 -> [w378 _]
              frame True {
                n170 = invoke class="VI" method="FP.Open"(reference=w379, error in=w380, "State"=w378) -> (error out=w381:errorcluster)  [unwired: 2 in, 4 out]
              }
              frame False {
              }
            }
          }
          frame "Maximize", "Maximized" {
            w383 = T4."Maximized" ("State")
            n171 = property class="VI"(reference=w387, error in=w389) -> (reference out=w386:refnum<vi>, error out=w388:errorcluster, "FP.State"=w385:T4)
            n172 = Not Equal?(x=w385, y=w383) -> (x != y?=w384:bool)
            n173 = case shown="True" w384 {
              tunnel: [w394 w395] -> w390
              tunnel: w388 -> [w393 w395]
              tunnel: w386 -> [w392 _]
              tunnel: w383 -> [w391 _]
              frame True {
                n174 = invoke class="VI" method="FP.Open"(reference=w392, error in=w393, "State"=w391) -> (error out=w394:errorcluster)  [unwired: 2 in, 4 out]
              }
              frame False {
              }
            }
          }
        }
        n175 = call "Enqueue Multiple States.vi"("queue in"=w325) -> ()  [unwired: 14 in, 1 out]
      }
      frame "UI: Get Preset Names" {
        n176 = Unbundle By Name(w397) -> ("Config"=w398:T6)
        n177 = call <vilib>:"Get Section Names.vi"("error in (no error)"=w400, "refnum"=w398) -> ("error out"=w399:errorcluster, "section names"=w396:string[])  [unwired: 7 in, 1 out]
        n178 = property on="Preset Name" class="CmbBox"("Strings[]"=w396) -> ()  [unwired: 2 in, 2 out]
      }
      frame "UI: Listen" {
        n179 = Unbundle By Name(w416) -> ("Hotkey"=w401:T8, "Keyboard"=w415:refnum<k1>)
        n180 = call "Stall Data Flow.vim"("value in"=w415, "milliseconds to wait"=u32 1) -> ("value out"=w406:refnum<k1>)  [unwired: 1 out]
        n181 = call-poly <vilib>:"Acquire Input Data.vi"("device ID"=w406, "error in (no error)"=w414) -> ("keys pressed"=w412:T8, "error out"=w413:errorcluster)  [unwired: 15 in, 1 out]
        n182 = Sort 1D Array(array=w412) -> (sorted array=w411:T8)
        n183 = Equal?(x=w401, y=w411) -> (x = y?=w410:bool)
        n184 = Select(t="Stats: Apply Preset\n", s=w410, f="") -> (s? t:f=w404:string)
        n185 = Concatenate Strings(w404, "UI: Listen" ("string")) -> (w402:string)
        n186 = call "Enqueue Multiple States.vi"("queue in"=w407, "State(s) at Back"=w402) -> ()  [unwired: 13 in, 1 out]
      }
      frame "---------- Macro ----------" {
        # "Do not put any code in this frame.\n(It is a separator no-op. You can make a copy of this frame to create a new Macro frame)"
        n187 = call "Enqueue Multiple States.vi"("queue in"=w417) -> ()  [unwired: 14 in, 1 out]
      }
      frame "Macro: Initialize" {
        w421 = "Data: Initialize\nInitialize Core Data\nData: Open Config\nUI: Get Preset Names\nUI: Initialize\nUI: Front Panel State >> Open"  # Data: Initialize Initialize Core Data Data: Open Config UI: Get Preset Names UI: Initialize UI: Front Panel State >> Open
        # "Initialization Macro\n(This is called once, when the VI starts)"
        n188 = call "Enqueue Multiple States.vi"("State(s) at Front"=w421, "queue in"=w420) -> ()  [unwired: 13 in, 1 out]
      }
      frame "Macro: Listen" {
        n189 = case shown="\"Start\"" w426 {
          tunnel: ["Data: Flush Queue" "UI: Listen"] -> w424
          frame "Stop", Default {
          }
          frame "Start" {
          }
        }
        n190 = call "Enqueue Multiple States.vi"("queue in"=w427, "State(s) at Back"=w424) -> ()  [unwired: 13 in, 1 out]
      }
      frame "Macro: Exit" {
        # "Exit Macro\n(This is called once, when the VI exits)"
        n191 = Unbundle By Name(w438) -> ("Core.Close Panel on Exit?"=w437:bool)
        n192 = Select(t="UI: Front Panel State >> Close\n", s=w437, f="") -> (s? t:f=w433:string)
        n193 = Concatenate Strings(w433, "Data: Cleanup\nExit") -> (w431:string)
        n194 = call "Enqueue Multiple States.vi"("State(s) at Front"=w431, "queue in"=w434) -> ()  [unwired: 13 in, 1 out]
      }
      frame "---------- Stats ----------" {
        # "Template Separator\n(You can make a copy of, or modify, this frame)"
        n195 = call "Enqueue Multiple States.vi"("queue in"=w440) -> ()  [unwired: 14 in, 1 out]
      }
      frame "Stats: Recalculate" {
        n196 = local read "Levels Available"() -> (w448:i32)
        n197 = local read "Dump Stat"() -> (w447:T1)
        n198 = local read "Levels"() -> (w449:T2)
        n199 = call "Recalculate Stats.vi"("Dump Stat"=w447, "Levels Available"=w448, "Levels"=w449) -> ("Levels Remaining"=→"Levels Remaining":i32, "Levels out"=w445:T2, "Valid?"=w444:bool)  [unwired: 6 in]
        n200 = call-poly <userlib>:"MGI Gray if.vi"("Boolean"=w444) -> ("Disabled"=w443:T3)
        n201 = property on="Start/Stop" class="Bool (strict)"("DisabledEnum"=w443) -> ()  [unwired: 2 in, 2 out]
        n202 = local write "Levels"(w445) -> ()
        n203 = call "Enqueue Multiple States.vi"("queue in"=w450) -> ()  [unwired: 14 in, 1 out]
      }
      frame "Stats: Apply Preset" {
        n204 = Unbundle By Name(w456) -> ("Res"=w455:cluster{"V":i16, "H":i16}[])
        n205 = local read "Levels"() -> (w454:T2)
        n206 = call "Perform Auto-Click.vi"("No Oxy?"="No Oxy Stat?", "error in (no error)"=w459, "Monitor Resolutions"=w455, "Monitor"="Select Monitor", "Levels"=w454) -> ("error out"=w458:errorcluster)  [unwired: 6 in]
      }
    }
  }
  n207 = Merge Errors(w9, w8) -> (w10:errorcluster)
  n208 = Release Queue(queue=w11, error in (no error)=w10) -> (error out=→"error out":errorcluster)  [unwired: 1 in, 2 out]
